vi "ErrorStringAndLog.vi"(8 "error in (no error)":errorcluster, 11 "Error":errorcluster) -> (0 "error out":errorcluster, 3 "Error String":string)   [LabVIEW 2012]
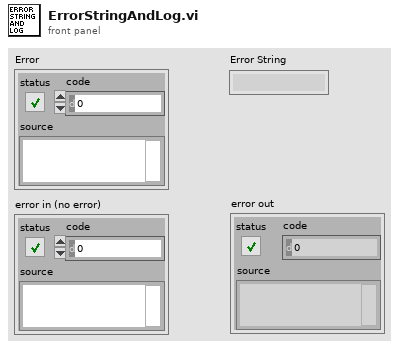
[diagram p1: front panel]
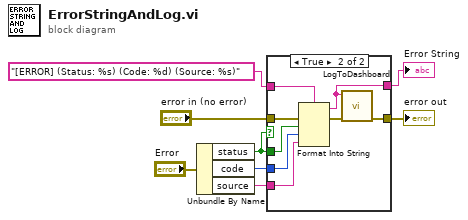
[diagram p0: block diagram]
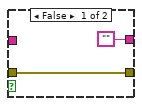
[diagram p2: hidden frame]
diagram:
  n1 = Unbundle By Name("Error") -> ("status"=w3:bool, "code"=w6:i32, "source"=w5:string)
  n2 = case shown="True" w3 {
    tunnel: ["" w18] -> w7
    tunnel: w3 -> [_ w16]
    tunnel: w6 -> [_ w15]
    tunnel: w5 -> [_ w14]
    tunnel: "[ERROR] (Status: %s) (Code: %d) (Source: %s)" ("format string") -> [_ w13]
    tunnel: [w9 w12] -> w2
    tunnel: "error in (no error)" -> [w9 w11]
    frame False {
    }
    frame True {
      n3 = Format Into String(format string=w13, error in=w11, w16, w15, w14) -> (resulting string=w18:string, error out=w17:errorcluster)  [unwired: 1 in]
      n4 = call "LogToDashboard.vi"("error in (no error)"=w17, "Info"=w18) -> ("error out"=w12:errorcluster)  [unwired: 9 in]
    }
  }
  "Error String" <- w7
  "error out" <- w2
